vi "CreatCom.vi"(8 "error in (no error)":errorcluster, 10 "file path (dialog if empty)":path=path "C:/AVC-BarCode/Setting Data/Com.ini", 11 "Data In":T1) -> (0 "error out":errorcluster, 3 "Data Out":T1)   [LabVIEW 2014]
uses:
  controls/Data.ctl
panel:
  out "element":string
  # "日期"
  # "機種名稱"
  # "機種代號"
  # "商品條碼"
  # "台"
  # "OK"
  # "NG"
  # "台"
  # "總計"
  # "台"
  # "日期"
  # "機種名稱"
  # "機種代號"
  # "商品條碼"
  # "台"
  # "OK"
  # "NG"
  # "台"
  # "總計"
  # "台"
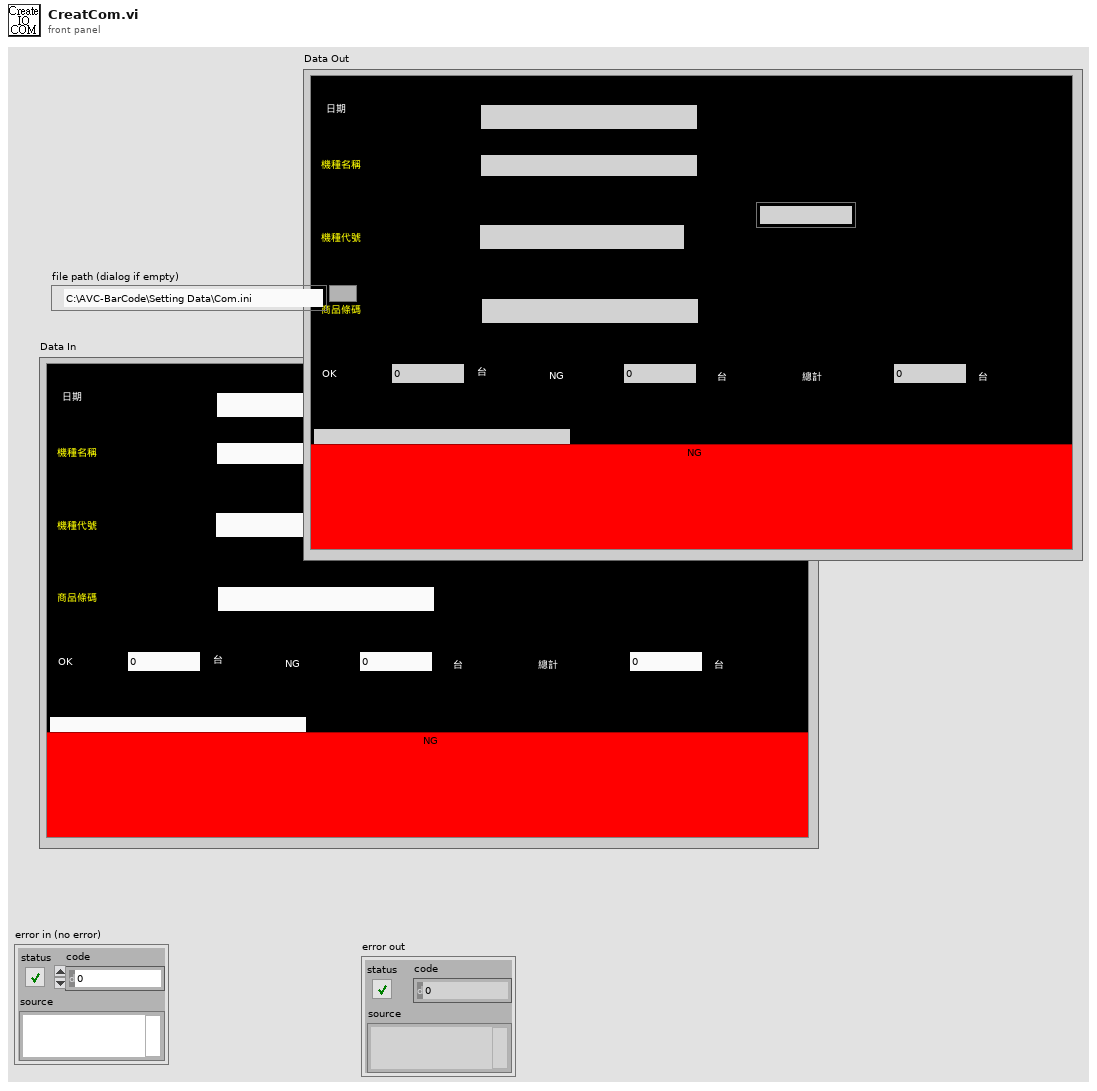
[diagram p1: front panel]
types:
  T1 = typedef "Data.ctl" = cluster{"Date":string, "BarCode1":string, "BarCode2":string, "BarCode3":string, "Message":string, "OK Count":u16, "NG Count":u16, "Total Count":u16, "ModelData":string[][], "OK&NG":bool, "COM1":refnum<visa-resource-name>, "COM2":refnum<visa-resource-name>, "IO":i32, "Time":u32, "TCP":refnum<k5>, "TCP 2":refnum<k5>, "COM3":refnum<visa-resource-name>}
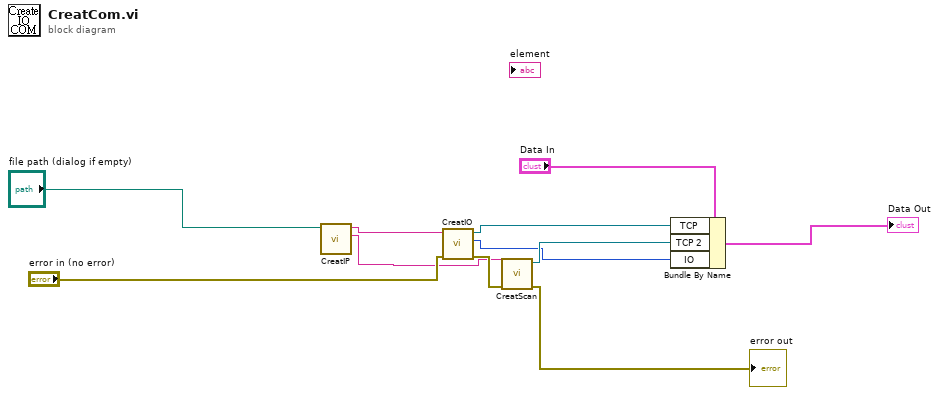
[diagram p0: block diagram]
diagram:
  n1 = call "CreatIP.vi"("file Path"="file path (dialog if empty)") -> ("Scan IP"=w2:string, "IO IP"=w3:string)  [unwired: 7 in, 2 out]
  n2 = call "CreatIO.vi"("error in (no error)"="error in (no error)", "address"=w3) -> ("error out"=w7:errorcluster, "IO"=w1:i32, "TCP Out"=w9:refnum<k5>)  [unwired: 7 in]
  n3 = call "CreatScan.vi"("error in (no error)"=w7, "address"=w2) -> ("error out"=→"error out":errorcluster, "TCP Out"=w6:refnum<k5>)  [unwired: 7 in, 1 out]
  n4 = Bundle By Name(cluster="Data In", "TCP"=w9, "TCP 2"=w6, "IO"=w1) -> (→"Data Out":T1)
